vi "Common Compose Setpoints.vi"(8 "Selected Correctors":u32[](array[numeric]), 9 "Corrector Kick Vector Manual Setpoint in":dbl[](array[numeric]), 10 "Corrector Kick Deltas Subset":dbl[](array[numeric]), 11 "Corrector Kick Vector in":dbl[](array[numeric])) -> (3 "Corrector Kicks":dbl[](array[numeric]))   [LabVIEW 2011, in "Common VIs.lvlib"]
doc: "Selects from the complete corrector kick vector (variation vector) the corrector kicks which are being used to FOFB. The unused correctors receives 0."
uses:
  Common VIs.lvlib
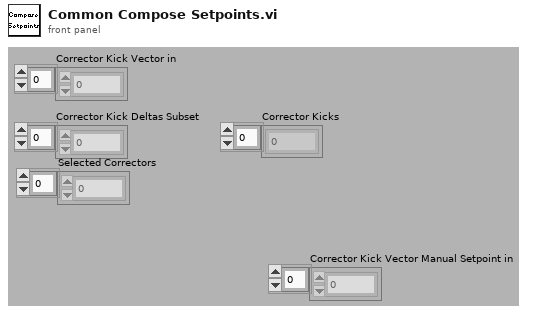
[diagram p1: front panel]
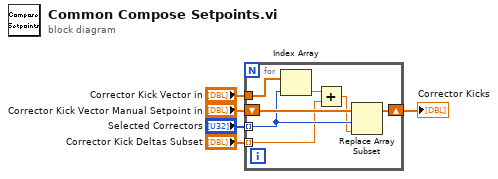
[diagram p0: block diagram]
diagram:
  n1 = for {
    tunnel: "Corrector Kick Deltas Subset" -> [w8] mode=indexing
    tunnel: "Selected Correctors" -> [w10] mode=indexing
    shift-right: [w12] -> w4
    shift-left: "Corrector Kick Vector Manual Setpoint in" -> [w11]
    tunnel: "Corrector Kick Vector in" -> [w6]
    n2 = Index Array(array=w6, index=w10) -> (element=w9:dbl)
    n3 = Add(x=w9, y=w8) -> (x+y=w7:dbl)
    n4 = Replace Array Subset(array=w11, new element=w7, index=w10) -> (w12:dbl[])
  }
  "Corrector Kicks" <- w4
